vi "SendPacket.vi"(10 "Input":string) -> ()   [LabVIEW 2014]
panel:
  # "For non-logging uses"
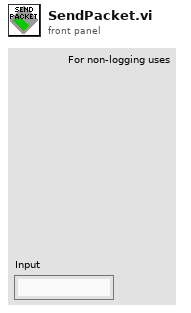
[diagram p1: front panel]
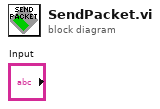
[diagram p0: block diagram]
diagram:
